vi "Main.vi"(11 "Module Admin":refnum<class "Delacor_lib_QMH_Module Admin.lvclass">) -> ()   [LabVIEW 2019, in "UI.lvlib"]
doc: "This template is based off of the Queued Message Handler design pattern and the Queued Message Handler project template that ships with LabVIEW.\n\nThe main difference is that the queue is private to this module and communication between modules is performed via Broadcast and Request events.\n\nRequest events are wrapped in public API methods and are handled in the Event Handling Loop (EHL) of this VI. Any module can register for Broadcast events sent by this module. The EHL generates messages based on user interface actions.\n\nThe Message Handling Loop (MHL) processes messages generated by the EHL, or by other messages. The messages are string values, so new messages can be added easily to the Message Cases case structure in the MHL. Each message cluster can also provide an optional value for Message Data, which is a variant that can be converted to whatever message-specific data is required.\n_____\nBased on Delacor QMH Project Template 5.0.0.82."
uses:
  UI.lvlib
  <vilib>/Delacor/Delacor QMH/Libraries/Module Admin_class/Delacor_lib_QMH_Module Admin.lvclass
  Module Data--cluster.ctl
  Stop Argument--cluster.ctl
  <vilib>/Delacor/Delacor QMH/Libraries/Message Queue_class/Delacor_lib_QMH_Message Queue.lvclass/Delacor_lib_QMH_Message Queue.ctl
  <vilib>/Delacor/Delacor QMH/Libraries/Module Admin_class/Delacor_lib_QMH_Module Admin.lvclass/Delacor_lib_QMH_Module Admin.ctl
  <vilib>/Utility/miscctls.llb/LVPointTypeDef.ctl
  <vilib>/Delacor/Delacor QMH/Libraries/Message Queue_class/Delacor_lib_QMH_Enqueue Message (Single).vi
  <vilib>/Delacor/Delacor QMH/Libraries/Module Admin_class/Delacor_lib_QMH_Get External Launch.vi
  <vilib>/Utility/error.llb/Error Cluster From Error Code.vi
  <vilib>/ErrorRing/Error Ring.xnode
  <vilib>/Delacor/Delacor QMH/Libraries/Message Queue_class/Delacor_lib_QMH_Message Queue.lvclass
  Adquisiion2/Adquisiion2.lvlib
  Config/Config.lvlib
  logging/logging.lvlib
panel:
  in  "config":bool
  in  "Stop":bool
  in  "Start":bool
  out "error out":errorcluster
  out "Status":string
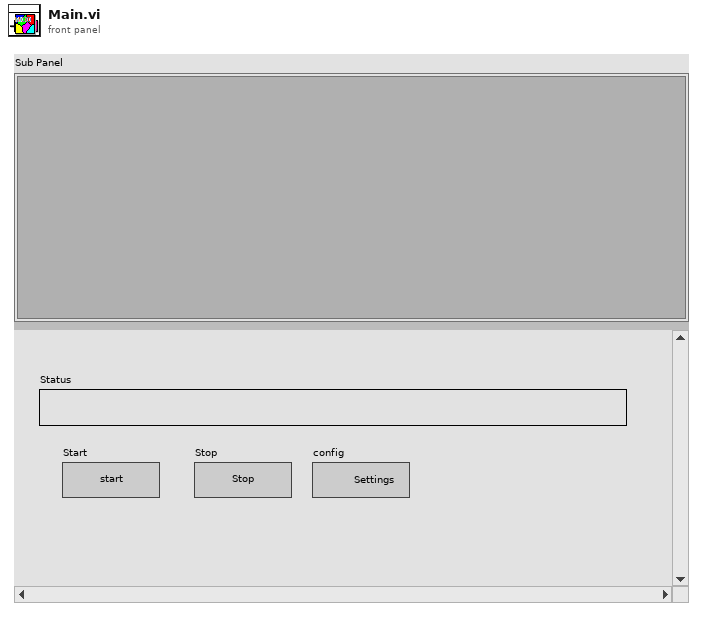
[diagram p1: front panel]
types:
  T1 = typedef "UI.lvlib/Request Events--cluster.ctl" = cluster{"Stop Module":refnum<user-event>, "Show Panel":refnum<user-event>, "Hide Panel":refnum<user-event>, "Get Module Execution Status":refnum<user-event>, "Show Diagram":refnum<user-event>}
  T2 = typedef "Config.lvlib/Broadcast Events--cluster.ctl" = cluster{"Module Did Init":refnum<user-event>, "Status Updated":refnum<user-event>, "Error Reported":refnum<user-event>, "Module Did Stop":refnum<user-event>, "Update Module Execution Status":refnum<user-event>}
  T3 = typedef "Adquisiion2.lvlib/Broadcast Events--cluster.ctl" = cluster{"Module Did Init":refnum<user-event>, "Status Updated":refnum<user-event>, "Error Reported":refnum<user-event>, "Module Did Stop":refnum<user-event>, "Update Module Execution Status":refnum<user-event>}
  T4 = typedef "logging.lvlib/Broadcast Events--cluster.ctl" = cluster{"Module Did Init":refnum<user-event>, "Status Updated":refnum<user-event>, "Error Reported":refnum<user-event>, "Module Did Stop":refnum<user-event>, "Update Module Execution Status":refnum<user-event>}
  T5 = typedef "UI.lvlib/Module Data--cluster.ctl" = cluster{"Status":string}
  T6 = enum32{"invalid lock state", "Not Locked", "Locked (No Password)", "Password-protected"}
  T7 = typedef "UI.lvlib/Stop Argument--cluster.ctl" = cluster{"Origin":string, "Exit via Stop Module Req?":bool, "Wait for Module to stop?":bool}
  T8 = enum32{"Invalid", "Standard", "Closed", "Hidden", "Minimized", "Maximized"}
  T9 = typedef "LVPointTypeDef.ctl" = cluster{"Horizontal":i16, "Vertical":i16}
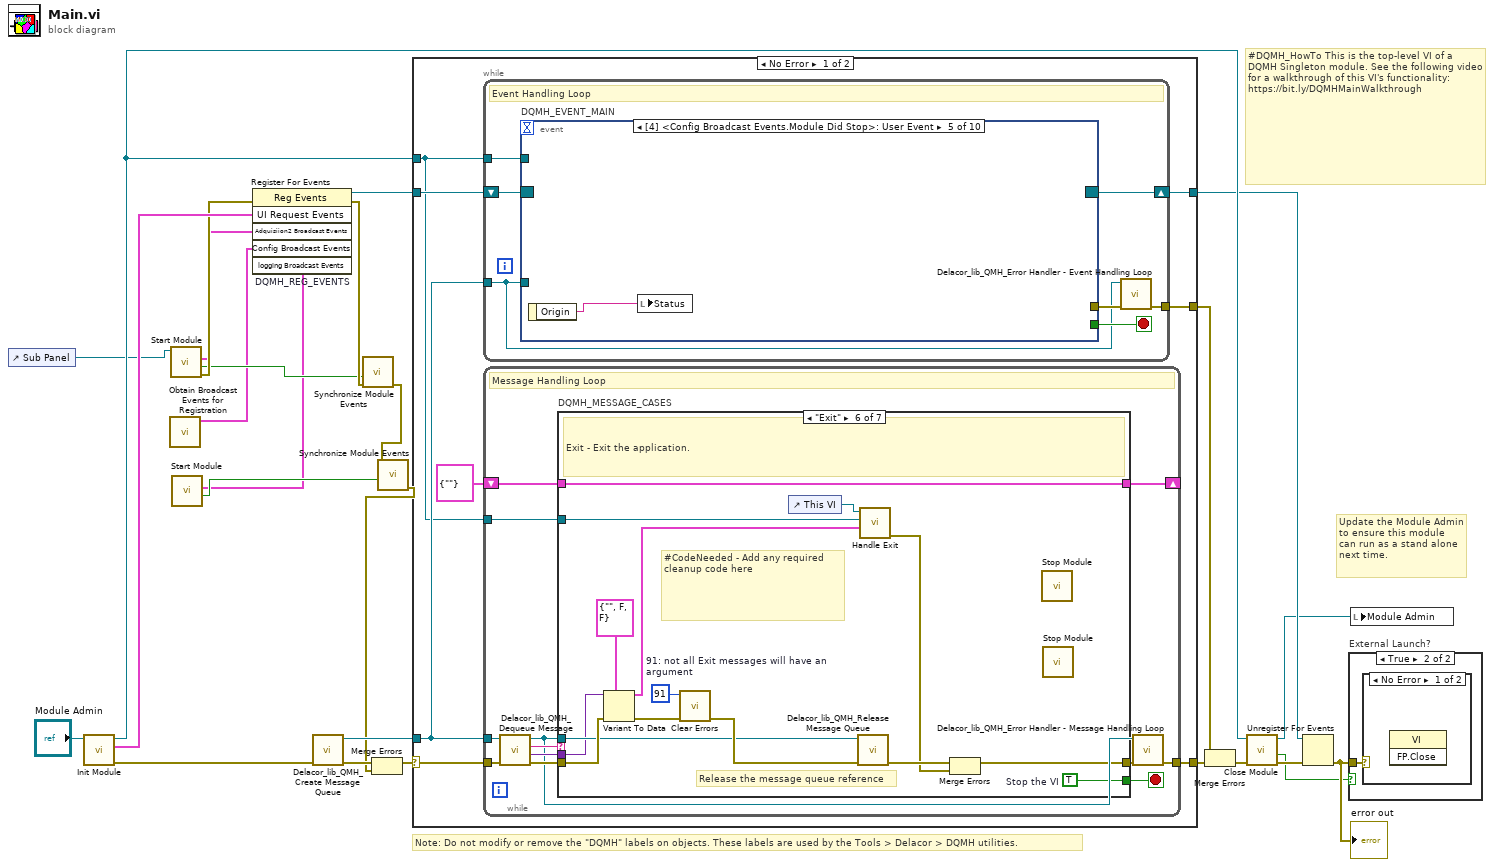
[diagram p0: block diagram]
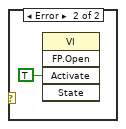
[diagram p3: hidden frame]
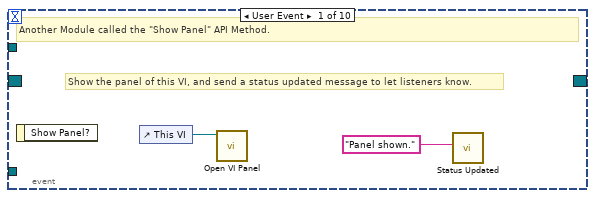
[diagram p4: hidden frame]
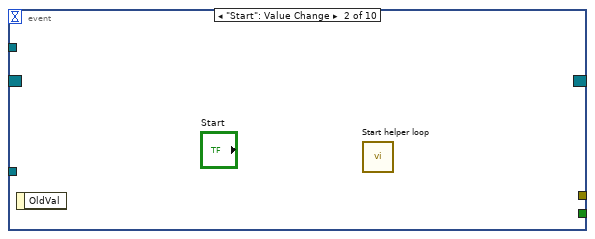
[diagram p5: hidden frame]
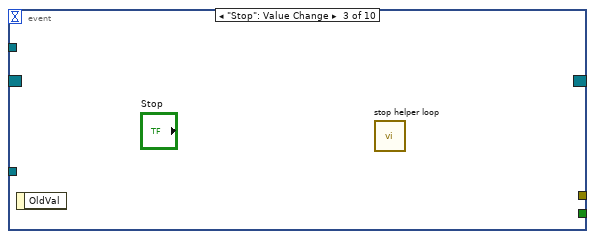
[diagram p6: hidden frame]
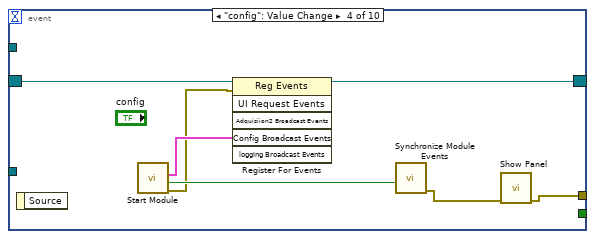
[diagram p7: hidden frame]
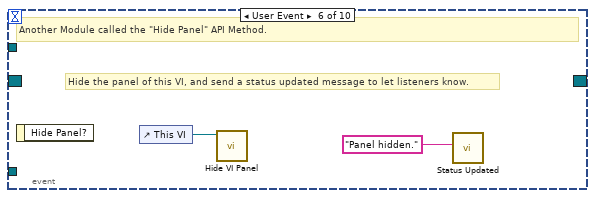
[diagram p8: hidden frame]
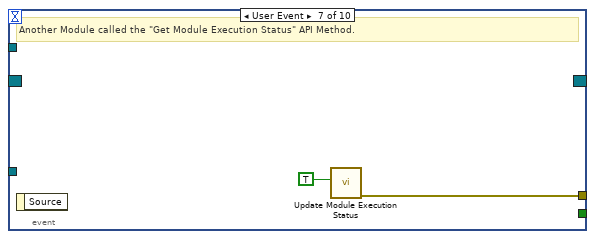
[diagram p9: hidden frame]
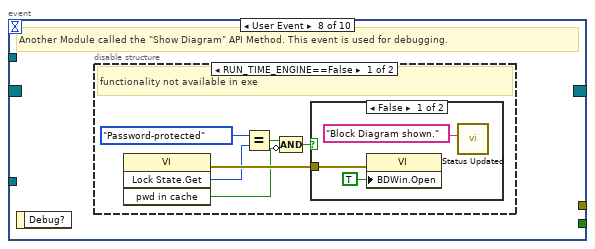
[diagram p10: hidden frame]
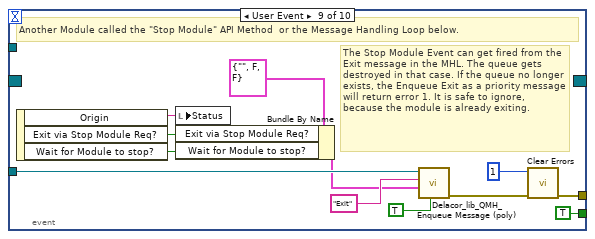
[diagram p13: hidden frame]
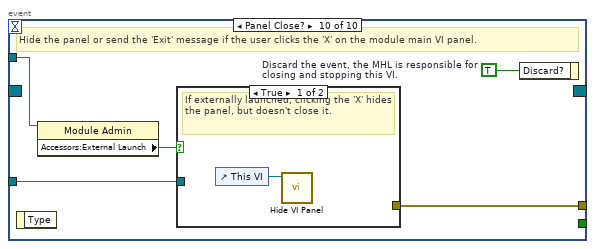
[diagram p14: hidden frame]
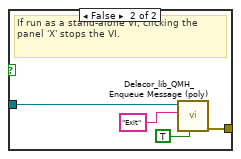
[diagram p15: hidden frame]
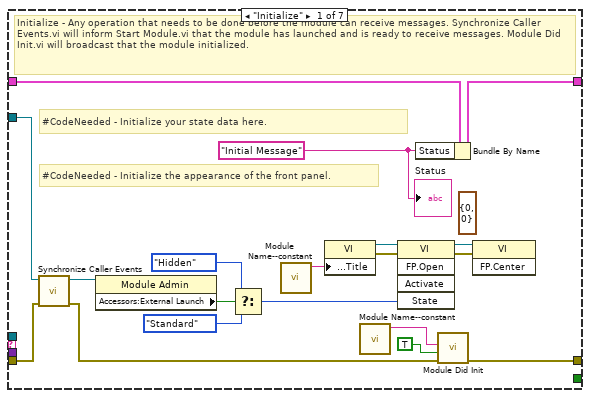
[diagram p16: hidden frame]
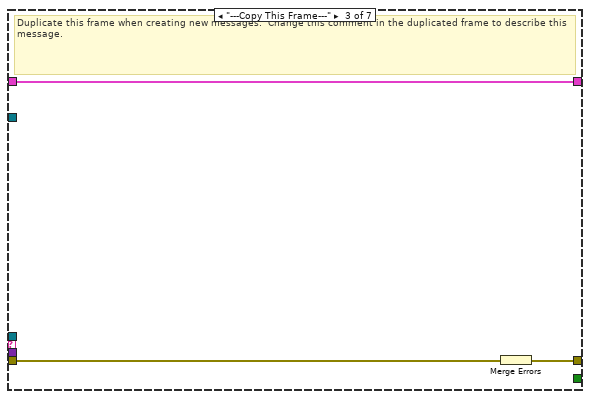
[diagram p18: hidden frame]
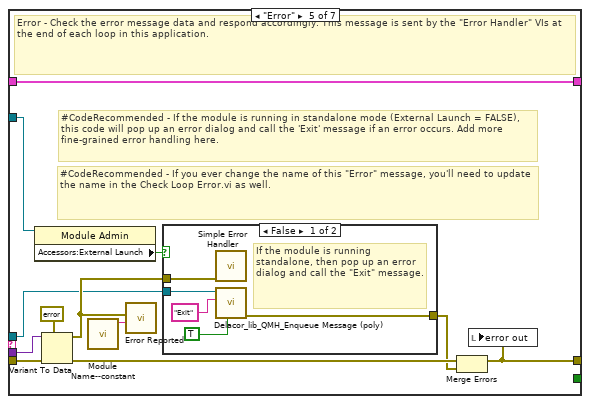
[diagram p20: hidden frame]
diagram:
  # "#DQMH_HowTo This is the top-level VI of a DQMH Singleton module. See the following video for a walkthrough of this VI's functionality: https://bit.ly/DQMHMainWalkthrough"
  # "Note: Do not modify or remove the \"DQMH\" labels on objects. These labels are used by the Tools > Delacor > DQMH utilities."
  # "Update the Module Admin to ensure this module can run as a stand alone next time."
  n1 = control-ref of="Sub Panel"() -> (w9:refnum<vi>)
  n2 = call "Init Module.vi"("Singleton Module Admin in"="Module Admin") -> ("error out"=w25:errorcluster, "UI Request Events"=w15:T1, "Singleton Module Admin out"=w18:refnum<class "Delacor_lib_QMH_Module Admin.lvclass">)  [unwired: 8 in]
  n3 = call "Obtain Broadcast Events for Registration.vi"() -> ("Config Broadcast Events"=w5:T2)  [unwired: 9 in, 2 out]
  n4 = call "Start Module.vi"("acqpanel"=w9) -> ("error out"=w10:errorcluster, "Wait for Event Sync?"=w6:bool, "Adquisiion2 Broadcast Events"=w8:T3)  [unwired: 7 in, 1 out]
  n5 = call "Start Module.vi"() -> ("Wait for Event Sync?"=w2:bool, "logging Broadcast Events"=w1:T4)  [unwired: 8 in, 2 out]
  n6 = register-events "DQMH_REG_EVENTS"(error in=w10, w15, w8, w5, w1) -> (reference out=w16:refnum<event-registration>, error out=w7:errorcluster)  [unwired: 1 in]
  n7 = call <vilib>:"Delacor_lib_QMH_Create Message Queue.vi"("error in (no error)"=w25) -> ("error out"=w20:errorcluster, "Message Queue"=w14:refnum<class "Delacor_lib_QMH_Message Queue.lvclass">)  [unwired: 9 in]
  n8 = call "Synchronize Module Events.vi"("error in (no error)"=w7, "Wait for Event Sync?"=w6) -> ("error out"=w4:errorcluster)  [unwired: 9 in]
  n9 = call "Synchronize Module Events.vi"("error in (no error)"=w4, "Wait for Event Sync?"=w2) -> ("error out"=w3:errorcluster)  [unwired: 9 in]
  n10 = Merge Errors(w20, w3) -> (w19:errorcluster)
  n11 = case shown="No Error" w19 {
    selector: w19 -> [w32 w173]
    tunnel: [w34 w172] -> w26
    tunnel: [w31 w178] -> w17
    tunnel: w16 -> [w29 w178]
    tunnel: w14 -> [w28 w171]
    tunnel: [w33 _] -> w23
    tunnel: w18 -> [w27 w174]
    frame No Error {
      n12 = while {
        tunnel: w28 -> [w35]
        shift-right: [w38] -> w31
        shift-left: w29 -> [w39]
        tunnel: [w40] -> w33
        tunnel: w27 -> [w36]
        stop <- w37 stop-if-true
        # "Event Handling Loop"
        n13 = event "DQMH_EVENT_MAIN" shown="[4] <Config Broadcast Events.Module Did Stop>: User Event" {
          selector: w39 -> [_ _ _ w50 _ _ _ _ _ _]
          dyn-events: [_ _ _ w49 _ _ _ _ _ _] -> w38
          timeout: _ -> [_ _ _ _ _ _ _ _ _ _]
          tunnel: [_ _ _ _ _ _ _ _ TRUE ("Discard?") _] -> w37
          tunnel: w35 -> [_ _ _ _ _ _ _ _ w72 w79]
          tunnel: [_ _ _ w44 _ _ w55 _ w75 w81] -> w41
          tunnel: w36 -> [_ _ _ _ _ _ _ _ _ w78]
          event User Event {
            # "Show the panel of this VI, and send a status updated message to let listeners know."
            # "Another Module called the \"Show Panel\" API Method."
            n14 = event-data() -> ()  [unwired: 1 in, 1 out]
            n15 = control-ref of="This VI"() -> (w43:refnum<vi>)
            n16 = call "Open VI Panel.vi"("VI"=w43) -> ()  [unwired: 10 in, 1 out]
            n17 = call "Status Updated.vi"("Status"="Panel shown." ("format string")) -> ()  [unwired: 10 in, 1 out]
          }
          event "Start": Value Change {
            n18 = event-data() -> ()  [unwired: 1 in, 1 out]
            n19 = call "Start helper loop.vi"() -> ()  [unwired: 11 in, 1 out]
          }
          event "Stop": Value Change {
            n20 = event-data() -> ()  [unwired: 1 in, 1 out]
            n21 = call "stop helper loop.vi"() -> ()  [unwired: 11 in, 1 out]
          }
          event "config": Value Change {
            n22 = event-data() -> ()  [unwired: 1 in, 1 out]
            n23 = call "Start Module.vi"() -> ("error out"=w46:errorcluster, "Wait for Event Sync?"=w47:bool, "Config Broadcast Events"=w48:T2)  [unwired: 8 in, 1 out]
            n24 = register-events(reference=w50, error in=w46, w48) -> (reference out=w49:refnum<event-registration>)  [unwired: 3 in, 1 out]
            n25 = call "Synchronize Module Events.vi"("Wait for Event Sync?"=w47) -> ("error out"=w45:errorcluster)  [unwired: 10 in]
            n26 = call "Show Panel.vi"("error in (no error)"=w45) -> ("error out"=w44:errorcluster)  [unwired: 10 in]
          }
          event User Event {
            n27 = event-data() -> ("Origin"=w51:string)  [unwired: 1 in]
            n28 = local write "Status"(w51) -> ()
          }
          event User Event {
            # "Hide the panel of this VI, and send a status updated message to let listeners know."
            # "Another Module called the \"Hide Panel\" API Method."
            n29 = event-data() -> ()  [unwired: 1 in, 1 out]
            n30 = control-ref of="This VI"() -> (w53:refnum<vi>)
            n31 = call "Hide VI Panel.vi"("VI"=w53) -> ()  [unwired: 10 in, 1 out]
            n32 = call "Status Updated.vi"("Status"="Panel hidden." ("format string")) -> ()  [unwired: 10 in, 1 out]
          }
          event User Event {
            # "Another Module called the \"Get Module Execution Status\" API Method."
            n33 = event-data() -> ()  [unwired: 1 in, 1 out]
            n34 = call "Update Module Execution Status.vi"("Running?"=TRUE) -> ("error out"=w55:errorcluster)  [unwired: 10 in]
          }
          event User Event {
            # "Another Module called the \"Show Diagram\" API Method. This event is used for debugging."
            n35 = event-data() -> ()  [unwired: 1 in, 1 out]
            n36 = disable-structure shown="RUN_TIME_ENGINE==False" {
              frame condition #0 (active) {
                # "functionality not available in exe"
                n37 = invoke class="VI" method="Lock State.Get"() -> (error out=w61:errorcluster, "Get Lock State"=w60:T6, "pwd in cache"=w57:bool)  [unwired: 4 in, 1 out]
                n38 = Equal?(x=T6."Password-protected", y=w60) -> (x = y?=w58:bool)
                n39 = Compound Arithmetic op=AND(w58, invert w57) -> (w56:bool)
                n40 = case shown="False" w56 {
                  tunnel: w61 -> [w64 _]
                  frame False {
                    n41 = property class="VI"(error in=w64, "BDWin.Open"=TRUE ("Block Diagram Window:Open")) -> ()  [unwired: 1 in, 2 out]
                    n42 = call "Status Updated.vi"("Status"="Block Diagram shown." ("format string")) -> ()  [unwired: 10 in, 1 out]
                  }
                  frame True {
                    # "Password-protected VI, and the password is not in the cache. Do not show the diagram."
                  }
                }
              }
              frame condition #1 {
              }
            }
          }
          event User Event {
            # "The Stop Module Event can get fired from the Exit message in the MHL. The queue gets destroyed in that case. If the queue no longer exists, the Enqueue Exit as a priority message will return error 1. It is safe to ignore, because the module is already exiting."
            # "Another Module called the \"Stop Module\" API Method  or the Message Handling Loop below."
            n43 = event-data() -> ("Origin"=w71:string, "Exit via Stop Module Req?"=w67:bool, "Wait for Module to stop?"=w66:bool)  [unwired: 1 in]
            n44 = local write "Status"(w71) -> ()
            n45 = Bundle By Name(cluster=T7 {"Origin"="", "Exit via Stop Module Req?"=FALSE, "Wait for Module to stop?"=FALSE} ("Stop Argument"), "Exit via Stop Module Req?"=w67, "Wait for Module to stop?"=w66) -> (w65:T7)
            n46 = call-poly <vilib>:"Delacor_lib_QMH_Enqueue Message (poly).vi"("Priority Message? (F)"=TRUE, "Message Data"=w65, "Message"="Exit", "Message Queue in"=w72) -> ("error out"=w76:errorcluster)  [unwired: 6 in, 1 out]
            n47 = call <vilib>:"Clear Errors.vi"("error in (no error)"=w76, "specific error code to clear (0: all)"=1) -> ("error out"=w75:errorcluster)  [unwired: 4 in, 1 out]
          }
          event Panel Close? {
            w80 = TRUE  # Discard the event, the MHL is responsible for closing and stopping this VI.
            # "Hide the panel or send the 'Exit' message if the user clicks the 'X' on the module main VI panel."
            n48 = event-data() -> ()  [unwired: 1 in, 1 out]
            n49 = property class="Module Admin"(reference=w78) -> ("Accessors:External Launch"=w77:bool)  [unwired: 1 in, 2 out]
            n50 = case shown="True" w77 {
              tunnel: w79 -> [_ w85]
              tunnel: [_ w86] -> w81
              frame True {
                # "If externally launched, clicking the 'X' hides the panel, but doesn't close it."
                n51 = control-ref of="This VI"() -> (w82:refnum<vi>)
                n52 = call "Hide VI Panel.vi"("VI"=w82) -> ()  [unwired: 10 in, 1 out]
              }
              frame False {
                # "If run as a stand-alone VI, clicking the panel 'X' stops the VI."
                n53 = call-poly <vilib>:"Delacor_lib_QMH_Enqueue Message (poly).vi"("Priority Message? (F)"=TRUE, "Message"="Exit", "Message Queue in"=w85) -> ("error out"=w86:errorcluster)  [unwired: 7 in, 1 out]
              }
            }
            n54 = event-data("Discard?"=w80) -> ()  [unwired: 1 in, 1 out]
          }
        }
        n55 = call-dynamic "Delacor_lib_QMH_Error Handler - Event Handling Loop.vi"("error in (no error)"=w41, "Message Queue in"=w35) -> ("dup error in"=w40:errorcluster)  [unwired: 8 in, 1 out]
      }
      n56 = while {
        tunnel: w28 -> [w89]
        shift-right: [w93] -> _
        shift-left: T5 {"Status"=""} ("Data Cluster") -> [w94]
        tunnel: w32 -> [w97]
        tunnel: [w95] -> w34
        tunnel: w27 -> [w87]
        stop <- w92 stop-if-true
        # "Message Handling Loop"
        n57 = call-dynamic "Delacor_lib_QMH_Dequeue Message.vi"("error in (no error)"=w97, "Message Queue in"=w89) -> ("error out"=w96:errorcluster, "Message Data"=w90:variant, "Message"=w91:string, "Message Queue out"=w88:refnum<class "Delacor_lib_QMH_Message Queue.lvclass">)  [unwired: 6 in]
        n58 = case "DQMH_MESSAGE_CASES" shown="\"Exit\"" w91 {
          selector: w91 -> [_ _ _ _ _ _ w158]
          tunnel: w88 -> [_ _ _ _ w128 w150 _]
          tunnel: w96 -> [w115 w119 w122 w124 w135 w156 w160]
          tunnel: [w113 w119 w121 w124 w131 w153 w161] -> w98
          tunnel: w94 -> [w104 w118 w120 w123 w130 w149 w159]
          tunnel: [w103 w118 w120 w123 w130 w149 w159] -> w93
          tunnel: [_ _ _ _ _ w148 _] -> w92
          tunnel: w90 -> [_ _ _ _ w129 w147 _]
          tunnel: w87 -> [w105 _ _ _ w127 w142 _]
          frame "Initialize" {
            (unwired) T9 {"Horizontal"=0, "Vertical"=0} ("Origin")
            w99 = "Initial Message" ("Initial Message")
            # "#CodeNeeded - Initialize the appearance of the front panel."
            # "#CodeNeeded - Initialize your state data here."
            # "Initialize - Any operation that needs to be done before the module can receive messages. Synchronize Caller Events.vi will inform Start Module.vi that the module has launched and is ready to receive messages. Module Did Init.vi will broadcast that the module initialized."
            n59 = call "Synchronize Caller Events.vi"("error in (no error)"=w115, "Singleton Module Admin in"=w105) -> ("error out"=w114:errorcluster, "Singleton Module Admin out"=w100:refnum<class "Delacor_lib_QMH_Module Admin.lvclass">)  [unwired: 8 in]
            n60 = property class="Module Admin"(reference=w100) -> ("Accessors:External Launch"=w109:bool)  [unwired: 1 in, 2 out]
            n61 = Select(t=T8."Hidden" ("State"), s=w109, f=T8."Standard" ("State")) -> (s? t:f=w106:T8)
            n62 = call "Module Name--constant.vi"() -> ("Module Name"=w112:string)  [unwired: 11 in]
            n63 = property class="VI"("Front Panel.Title"=w112) -> (reference out=w111:refnum<vi>, error out=w117:errorcluster)  [unwired: 2 in]
            n64 = call "Module Name--constant.vi"() -> ("Module Name"=w101:string)  [unwired: 11 in]
            n65 = invoke class="VI" method="FP.Open"(reference=w111, error in=w117, "State"=w106) -> (reference out=w110:refnum<vi>, error out=w116:errorcluster)  [unwired: 2 in, 3 out]
            n66 = Bundle By Name(cluster=w104, "Status"=w99) -> (w103:T5)
            n67 = call "Module Did Init.vi"("error in (no error)"=w114, "Initialized?"=TRUE, "Origin"=w101) -> ("error out"=w113:errorcluster)  [unwired: 8 in]
            n68 = invoke class="VI" method="FP.Center"(reference=w110, error in=w116) -> ()  [unwired: 1 in, 3 out]
            "Status" <- w99
          }
          frame "--- Module Specific ---" {
            # "Separator -- The following cases handle messages specific to this Module."
          }
          frame "---Copy This Frame---" {
            # "Duplicate this frame when creating new messages.  Change this comment in the duplicated frame to describe this message."
            n69 = Merge Errors(w122) -> (w121:errorcluster)
          }
          frame "--- Exit and Error Handling---" {
            # "Separator - The following cases handle errors and exit messages."
          }
          frame "Error" {
            # "#CodeRecommended - If you ever change the name of this \"Error\" message, you'll need to update the name in the Check Loop Error.vi as well."
            # "#CodeRecommended - If the module is running in standalone mode (External Launch = FALSE), this code will pop up an error dialog and call the 'Exit' message if an error occurs. Add more fine-grained error handling here."
            # "Error - Check the error message data and respond accordingly. This message is sent by the \"Error Handler\" VIs at the end of each loop in this application."
            n70 = property class="Module Admin"(reference=w127) -> ("Accessors:External Launch"=w126:bool)  [unwired: 1 in, 2 out]
            n71 = Variant To Data(error in=w135, type=errorcluster {"status"=FALSE, "code"=0, "source"=""} ("error constant"), Variant=w129) -> (data=w136:errorcluster, error out=w133:errorcluster)
            n72 = call "Module Name--constant.vi"() -> ("Module Name"=w125:string)  [unwired: 11 in]
            n73 = call "Error Reported.vi"("Additional Information"=w125, "Error"=w136) -> ()  [unwired: 9 in, 1 out]
            n74 = case shown="False" w126 {
              tunnel: [w141 _] -> w132
              tunnel: w128 -> [w139 _]
              tunnel: w136 -> [w140 _]
              frame False {
                # "If the module is running standalone, then pop up an error dialog and call the \"Exit\" message."
                n75 = call <vilib>:"Simple Error Handler.vi"("error in (no error)"=w140) -> ()  [unwired: 4 in, 5 out]
                n76 = call-poly <vilib>:"Delacor_lib_QMH_Enqueue Message (poly).vi"("Priority Message? (F)"=TRUE, "Message"="Exit", "Message Queue in"=w139) -> ("error out"=w141:errorcluster)  [unwired: 7 in, 1 out]
              }
              frame True {
                # "If the module was launched externally, calling the Error Reported broadcast VI is the only action performed by the \"Error\" message. The module's caller can then process the error appropriately."
              }
            }
            n77 = Merge Errors(w133, w132) -> (w131:errorcluster)
            n78 = local write "error out"(w131) -> ()
          }
          frame "Exit" {
            w146 = 91  # 91: not all Exit messages will have an argument
            w148 = TRUE  # Stop the VI
            # "Release the message queue reference"
            # "#CodeNeeded - Add any required cleanup code here"
            # "Exit - Exit the application."
            n79 = Variant To Data(error in=w156, type=T7 {"Origin"="", "Exit via Stop Module Req?"=FALSE, "Wait for Module to stop?"=FALSE} ("Stop Argument"), Variant=w147) -> (data=w144:T7, error out=w152:errorcluster)
            n80 = call <vilib>:"Clear Errors.vi"("error in (no error)"=w152, "specific error code to clear (0: all)"=w146) -> ("error out"=w155:errorcluster)  [unwired: 4 in, 1 out]
            n81 = control-ref of="This VI"() -> (w143:refnum<vi>)
            n82 = call-dynamic "Delacor_lib_QMH_Release Message Queue.vi"("error in (no error)"=w155, "Message Queue"=w150) -> ("error out"=w154:errorcluster)  [unwired: 9 in]
            n83 = call "Handle Exit.vi"("Stop Argument"=w144, "Admin in"=w142, "VI reference"=w143) -> ("error out"=w151:errorcluster)  [unwired: 7 in, 1 out]
            n84 = Merge Errors(w154, w151) -> (w153:errorcluster)
            n85 = call "Stop Module.vi"() -> ()  [unwired: 11 in, 1 out]
            n86 = call "Stop Module.vi"() -> ()  [unwired: 11 in, 1 out]
          }
          frame Default {
            # "'Default' case only runs if there is a message that isn't defined in any of the other cases.  Output a programming error."
            n87 = call "Module Name--constant.vi"() -> ("Module Name"=w157:string)  [unwired: 11 in]
            n88 = xnode "Error Ring"("parameter 0"=w158, "parameter 1"=w157) -> ("error out"=w162:errorcluster)
            n89 = Merge Errors(w160, w162) -> (w161:errorcluster)
          }
        }
        n90 = call-dynamic "Delacor_lib_QMH_Error Handler - Message Handling Loop.vi"("error in (no error)"=w98, "Message Queue in"=w88) -> ("dup error in"=w95:errorcluster)  [unwired: 8 in, 1 out]
      }
    }
    frame Error {
      # "Synchronize Caller Events.vi will inform Start Module.vi that the module has launched and will let the code calling Start Module.vi register for broadcasts and would permit the caller receive the broadcast that an error occurred at launch time."
      n91 = call-dynamic "Delacor_lib_QMH_Release Message Queue.vi"("error in (no error)"=w173, "Message Queue"=w171) -> ("error out"=w172:errorcluster)  [unwired: 9 in]
      n92 = call "Synchronize Caller Events.vi"("Singleton Module Admin in"=w174) -> ("error out"=w179:errorcluster)  [unwired: 9 in, 1 out]
      n93 = call "Module Name--constant.vi"() -> ("Module Name"=w177:string)  [unwired: 11 in]
      n94 = Format Into String(format string="An error occurred during initialization. %s is no longer running.", w177) -> (resulting string=w175:string)  [unwired: 2 in, 1 out]
      n95 = Merge Errors(w172, w179) -> (w180:errorcluster)
      n96 = call "Error Reported.vi"("Additional Information"=w175, "Error"=w180) -> ()  [unwired: 9 in, 1 out]
    }
  }
  n97 = Merge Errors(w23, w26) -> (w22:errorcluster)
  n98 = call "Close Module.vi"("error in (no error)"=w22, "Module Admin in"=w18) -> ("error out"=w24:errorcluster, "External Launch"=w11:bool, "Module Admin out"=w12:refnum<class "Delacor_lib_QMH_Module Admin.lvclass">)  [unwired: 7 in]
  n99 = Unregister For Events(event registration refnum=w17, error in=w24) -> (error out=w21:errorcluster)
  "error out" <- w21
  n100 = case "External Launch?" shown="True" w11 {
    tunnel: w21 -> [_ w181]
    frame False {
    }
    frame True {
      n101 = case shown="No Error" w181 {
        frame No Error {
          n102 = invoke class="VI" method="FP.Close"() -> ()  [unwired: 3 in, 3 out]
        }
        frame Error {
          n103 = invoke class="VI" method="FP.Open"("Activate"=TRUE ("Activate?")) -> ()  [unwired: 4 in, 5 out]
        }
      }
    }
  }
  n104 = local write "Module Admin"(w12) -> ()
